vi "NI-XNET Filter - Get All Names from Database.vi"(0 "database in (:memory:)":refnum<k21>=":memory:", 5 "error in (no error)":errorcluster, 6 "Filter Cluster":string) -> (10 "Number of Frames":i32[](array[numeric]), 12 "Number of Clusters":i32, 13 "Number of Signals":i32[][](array[numeric]), 14 "Clusters":string[](array[string]), 15 "Frames":string[][](array[string]), 16 "Signals":string[][][](array[string]), 19 "error out":errorcluster)   [LabVIEW 2020, in "Vires VTD System Explorer.lvlib"]
uses:
  Vires VTD System Explorer.lvlib
  <resource>/objmgr/xnet.rc
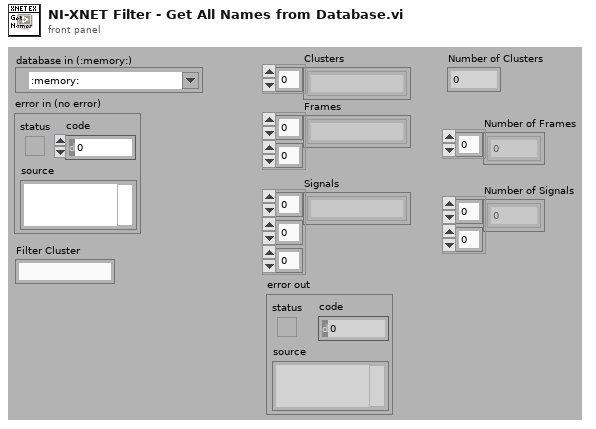
[diagram p1: front panel]
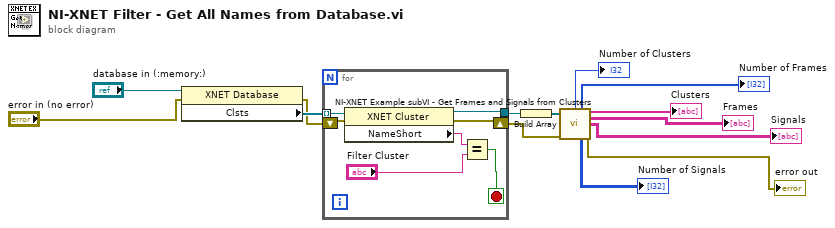
[diagram p0: block diagram]
diagram:
  n1 = property class="XNET Database"(reference="database in (:memory:)", error in="error in (no error)") -> (error out=w4:errorcluster, "Clsts"=w5:refnum<k21>[])  [unwired: 1 out]
  n2 = for {
    tunnel: w5 -> [w21] mode=indexing
    tunnel: [w20] -> w2
    shift-right: [w15] -> w3
    shift-left: w4 -> [w16]
    stop <- w19 stop-if-true
    n3 = property class="XNET Cluster"(reference=w21, error in=w16) -> (reference out=w20:refnum<k21>, error out=w15:errorcluster, "NameShort"=w18:string)
    n4 = Equal?(x=w18, y="Filter Cluster") -> (x = y?=w19:bool)
  }
  n5 = Build Array(w2) -> (w1:refnum<k21>[])
  n6 = call "NI-XNET Example subVI - Get Frames and Signals from Clusters.vi"("XNET Clusters"=w1, "error in"=w3) -> ("Number of Clusters"=→"Number of Clusters":i32, "Number of Frames"=→"Number of Frames":i32[], "Cluster Names"=→"Clusters":string[], "Frame Names"=→"Frames":string[][], "Signal Names"=→"Signals":string[][][], "Number of Signals"=→"Number of Signals":i32[][], "error out"=→"error out":errorcluster)  [unwired: 2 in, 5 out]
